vi "StartRecord.vi"(4 "error in (no error)":errorcluster, 6 "ClusterRefCtrlIN":T1, 7 "task/channels in":refnum<k21>) -> (0 "error out":errorcluster, 2 "RecStarted":bool, 3 "task out":refnum<k21>)   [LabVIEW 2017]
uses:
  <vilib>/DAQmx/write.llb/DAQmx Write (Digital Bool 1Line 1Point).vi
  DefDeType/ClusterRefCtrl.ctl
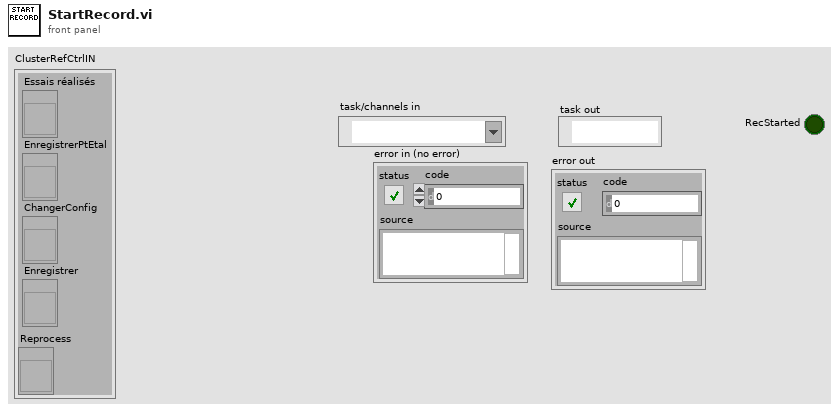
[diagram p1: front panel]
types:
  T1 = typedef "ClusterRefCtrl.ctl" = cluster{"Essais réalisés":refnum<vi>, "EnregistrerPtEtal":refnum<vi>, "ChangerConfig":refnum<vi>, "Enregistrer":refnum<vi>, "Reprocess":refnum<vi>}
  T2 = enum8{"Enabled", "Disabled", "Disabled and Grayed Out"}
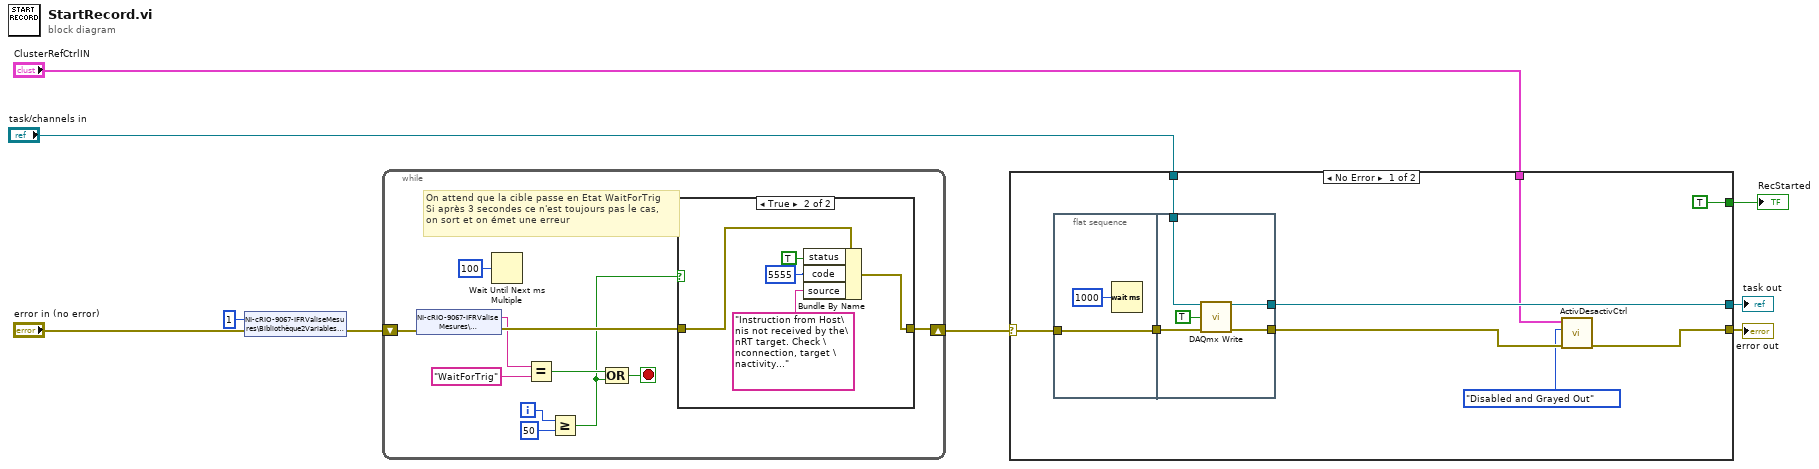
[diagram p0: block diagram]
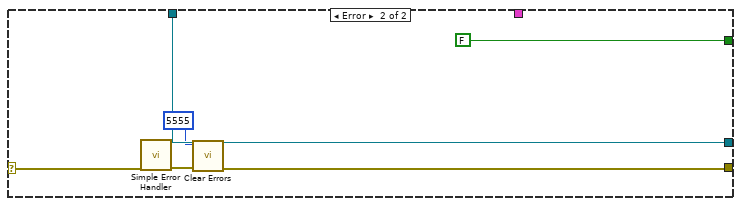
[diagram p2: hidden frame]
diagram:
  n1 = shared-variable "NI-cRIO-9067-IFRValiseMesures\\Bibliothèque2Variables.lvlib\\Instruction"(u8 1 ("Instruction"), error in="error in (no error)") -> (error out=w7:errorcluster)
  n2 = while {
    shift-right: [w11] -> w6
    shift-left: w7 -> [w20]
    i -> [w17]
    stop <- w14 stop-if-true
    # "On attend que la cible passe en Etat WaitForTrig\nSi après 3 secondes ce n'est toujours pas le cas, \non sort et on émet une erreur"
    n3 = shared-variable "NI-cRIO-9067-IFRValiseMesures\\Bibliothèque2Variables.lvlib\\RTState"(error in=w20) -> (w10:string, error out=w13:errorcluster)
    n4 = Wait Until Next ms Multiple(millisecond multiple=u32 100) -> ()  [unwired: 1 out]
    n5 = Equal?(x=w10, y="WaitForTrig") -> (x = y?=w15:bool)
    n6 = Greater Or Equal?(x=w17, y=50) -> (x >= y?=w12:bool)
    n7 = Compound Arithmetic op=OR(w15, w12) -> (w14:bool)
    n8 = case shown="True" w12 {
      tunnel: w13 -> [w21 w26]
      tunnel: [w21 w22] -> w11
      frame False {
      }
      frame True {
        n9 = Bundle By Name(cluster=w26, "status"=TRUE, "code"=5555, "source"="Instruction from Host\nis not received by the\nRT target. Check \nconnection, target \nactivity...") -> (w22:errorcluster)
      }
    }
  }
  n10 = case shown="No Error" w6 {
    selector: w6 -> [w35 w47]
    tunnel: "task/channels in" -> [w33 w48]
    tunnel: [w29 w44] -> w3
    tunnel: [w32 w48] -> w4
    tunnel: [TRUE ("RecStarted") FALSE ("RecStarted")] -> w2
    tunnel: "ClusterRefCtrlIN" -> [w28 _]
    frame No Error {
      n11 = flat-sequence {
        tunnel: w35 -> [w36]
        tunnel: [w36] -> w34
        tunnel: w34 -> [w41]
        tunnel: w33 -> [w39]
        tunnel: [w40] -> w30
        tunnel: [w38] -> w32
        frame #0 {
          n12 = Wait (ms)(milliseconds to wait=u32 1000) -> ()  [unwired: 1 out]
        }
        frame #1 {
          n13 = call-poly <vilib>:"DAQmx Write.vi"("task/channels in"=w39, "data"=TRUE, "error in"=w41) -> ("task out"=w38:refnum<k21>, "error out"=w40:errorcluster)  [unwired: 10 in, 1 out]
        }
      }
      n14 = call "ActivDesactivCtrl.vi"("error in (no error)"=w30, "Disabled"=T2."Disabled and Grayed Out", "Cluster"=w28) -> ("error out"=w29:errorcluster)  [unwired: 4 in]
    }
    frame Error {
      n15 = call <vilib>:"Simple Error Handler.vi"("error in (no error)"=w47) -> ("error out"=w46:errorcluster)  [unwired: 4 in, 4 out]
      n16 = call <vilib>:"Clear Errors.vi"("error in (no error)"=w46, "specific error code to clear (0: all)"=5555) -> ("error out"=w44:errorcluster)  [unwired: 4 in, 1 out]
    }
  }
  "task out" <- w4
  "error out" <- w3
  "RecStarted" <- w2
